vi "Labview_serial_arduino.vi"() -> ()   [LabVIEW 2022 SP3]
uses:
  <vilib>/Instr/_visa.llb/VISA Configure Serial Port (Instr).vi
panel:
  in  "Stop":bool
  out "Waveform Chart":cluster{dbl, dbl}(graph)
  out "error out":errorcluster
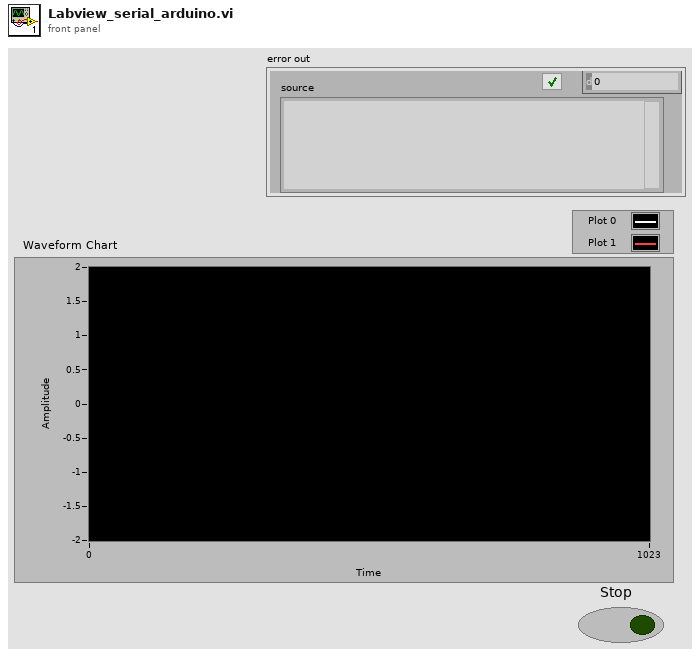
[diagram p1: front panel]
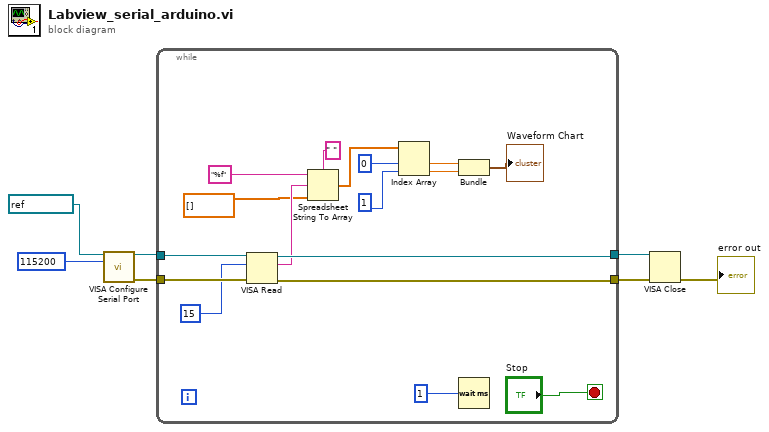
[diagram p0: block diagram]
diagram:
  n1 = call-poly "VISA Configure Serial Port"("VISA resource name"=refnum<visa-resource-name> "COM3", "baud rate (9600)"=u32 115200) -> ("VISA resource name out"=w5:refnum<visa-resource-name>, "error out"=w4:errorcluster)  [unwired: 12 in]
  n2 = while {
    tunnel: w5 -> [w24]
    tunnel: [w21] -> w3
    tunnel: w4 -> [w23]
    tunnel: [w22] -> w2
    stop <- "Stop" stop-if-true
    n3 = VISA Read(VISA resource name=w24, byte count=u32 15, error in (no error)=w23) -> (VISA resource name out=w21:refnum<visa-resource-name>, read buffer=w20:string, error out=w22:errorcluster)  [unwired: 1 out]
    n4 = Spreadsheet String To Array(delimiter (Tab)=" ", format string="%f", spreadsheet string=w20, array type (2D Dbl)=dbl[] []) -> (array=w12:dbl[])
    n5 = Index Array(array=w12, index #1=0 ("index"), index #2=1 ("index")) -> (element #1=w10:dbl, element #2=w9:dbl)
    n6 = Bundle(w10, w9) -> (→"Waveform Chart":cluster{dbl, dbl})  [unwired: 1 in]
    n7 = Wait (ms)(milliseconds to wait=u32 1) -> ()  [unwired: 1 out]
  }
  n8 = VISA Close(VISA resource name=w3, error in (no error)=w2) -> (error out=→"error out":errorcluster)
